vi "StartStop.vi"(8 "error in (no error)":errorcluster, 10 "Start/Stop":bool, 11 "Signal Generation in":refnum<class "Signal Generation.lvclass">) -> (0 "error out":errorcluster, 3 "Signal Generation out":refnum<class "Signal Generation.lvclass">)   [LabVIEW 2020, in "Signal Generation.lvlib" / "Signal Generation.lvclass"]
uses:
  Signal Generation.lvclass
  Signal Generation.lvclass/Signal Generation.ctl
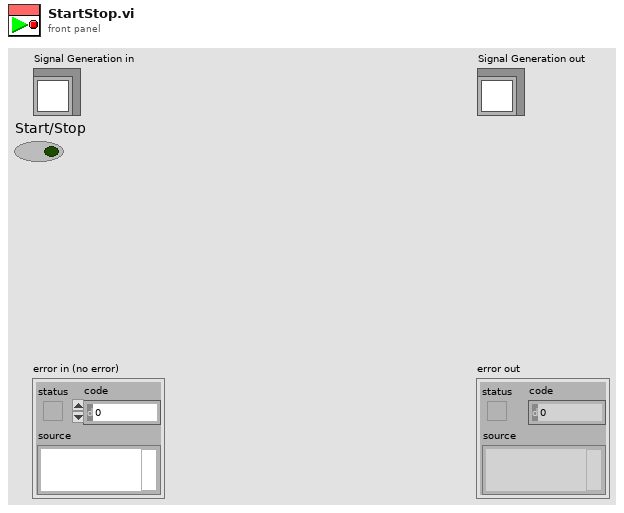
[diagram p1: front panel]
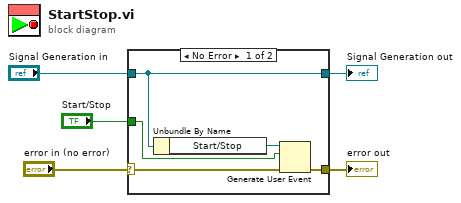
[diagram p0: block diagram]
diagram:
  n1 = case shown="No Error" "error in (no error)" {
    selector: "error in (no error)" -> [w8 w12]
    tunnel: [w7 w12] -> w4
    tunnel: [w10 w11] -> w2
    tunnel: "Signal Generation in" -> [w10 w11]
    tunnel: "Start/Stop" -> [w6 _]
    frame No Error {
      n2 = Unbundle By Name(w10) -> ("Start/Stop"=w9:refnum<user-event>)
      n3 = Generate User Event(user event=w9, event data cluster=w6, error in=w8) -> (error out=w7:errorcluster)  [unwired: 1 in, 1 out]
    }
    frame Error {
    }
  }
  "error out" <- w4
  "Signal Generation out" <- w2
